vi "ReadPoints.vi"(9 "Transform Points In":T2(array[cluster])) -> (1 "Transform Points out":T2(array[cluster]))   [LabVIEW 2017]
uses:
  ReadTextfileColumns.ctl
  AT901 API/Structures/Struct TransformationPoint.ctl
panel:
  in  "Skip Rows":i32
  in  "Abbrechen":bool
  in  "Column 4":T3
  in  "Column 3":T3
  in  "Column 2":T3
  in  "Column1":T3
  out "subarray":string[][](array[string])
  in  "Skip Lines":i32
  in  "stop":bool
  in  "Delimitor Strichpunkt":bool
  in  "Delimitor Leerzeichen":bool
  in  "DelimitorTab":bool
  in  "file path (use dialog)":path=path "C:/Users/Wehner/Desktop/Testfile.txt"
  # "Textfile Laden"
  # "Vorschau:"
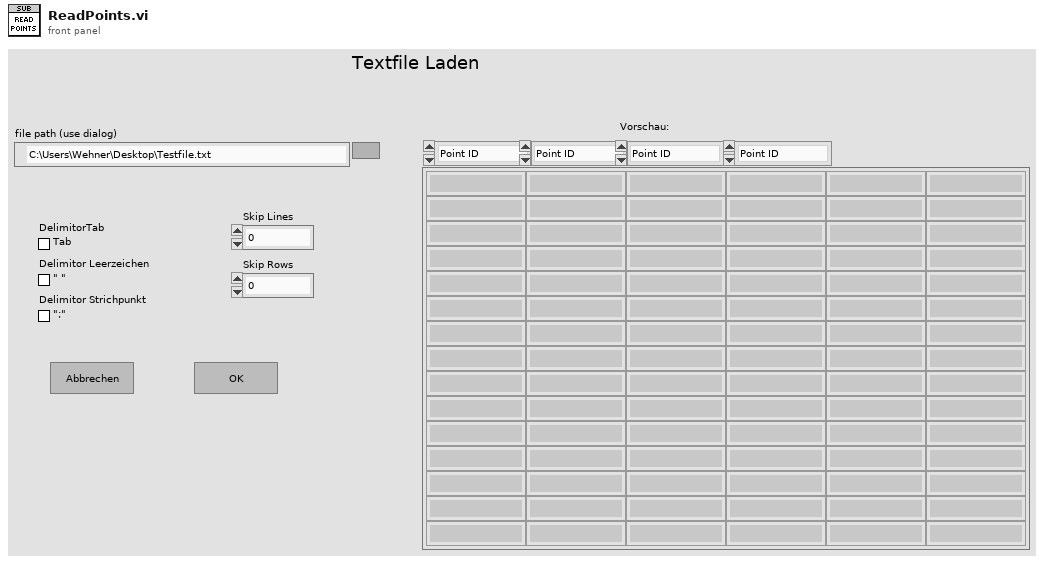
[diagram p1: front panel]
types:
  T1 = typedef "Struct TransformationPoint.ctl" = cluster{"dVal1":dbl, "dVal2":dbl, "dVal3":dbl, "dStd1":dbl, "dStd2":dbl, "dStd3":dbl, "dCovar12":dbl, "dCovar13":dbl, "dCovar23":dbl}
  T2 = cluster{"Punktnummer":string, "Transformation Point":T1}[]
  T3 = typedef "ReadTextfileColumns.ctl" = enum16{"Point ID", "X", "Y", "Z"}
  T4 = cluster{"Punktnummer":string, "Transformation Point":T1}
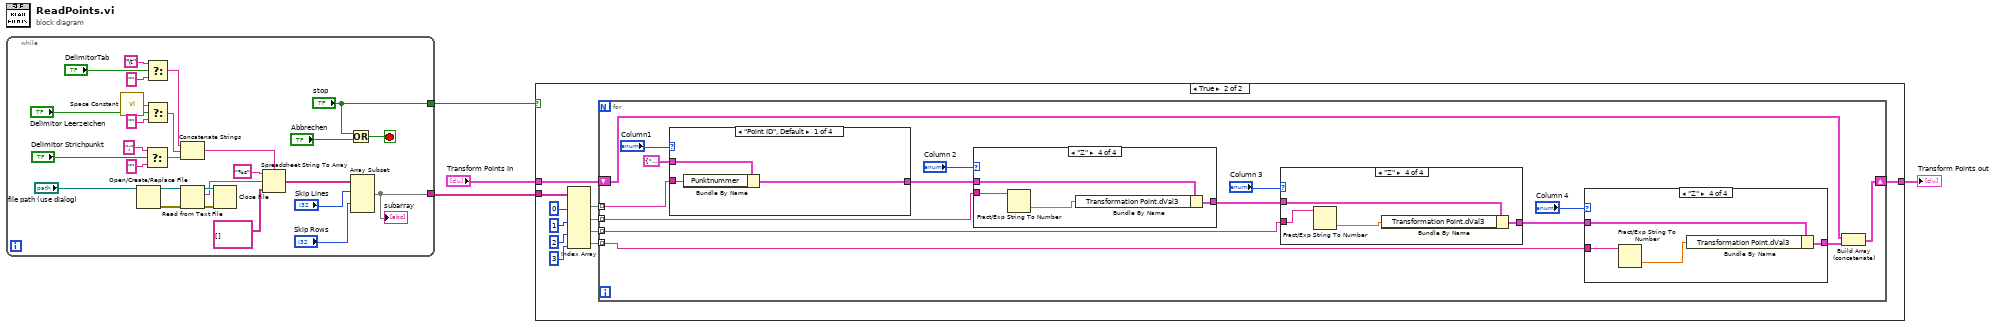
[diagram p0: block diagram]
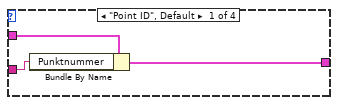
[diagram p3: hidden frame]
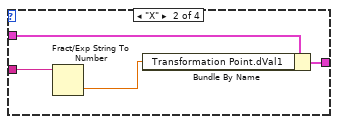
[diagram p4: hidden frame]
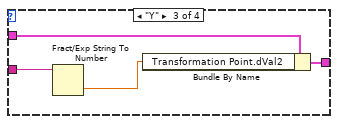
[diagram p5: hidden frame]
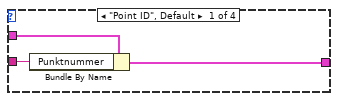
[diagram p6: hidden frame]
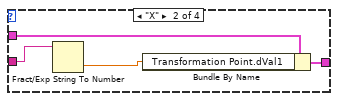
[diagram p7: hidden frame]
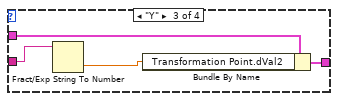
[diagram p8: hidden frame]
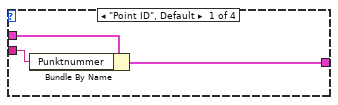
[diagram p9: hidden frame]
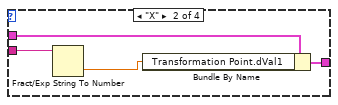
[diagram p10: hidden frame]
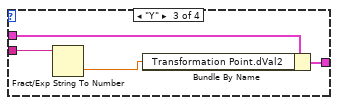
[diagram p11: hidden frame]
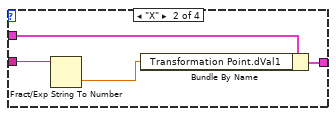
[diagram p12: hidden frame]
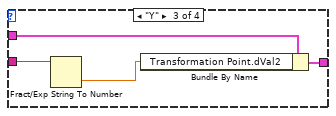
[diagram p13: hidden frame]
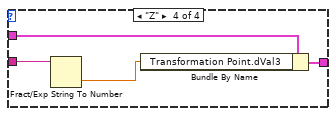
[diagram p14: hidden frame]
diagram:
  n1 = while {
    tunnel: [w15] -> w4
    tunnel: ["stop"] -> w3
    stop <- w13 stop-if-true
    n2 = call <vilib>:"Space Constant.vi"() -> ("String"=w23:string)
    n3 = Open/Create/Replace File(file path (use dialog)="file path (use dialog)") -> (refnum out=w8:refnum<file>, error out=w7:errorcluster)  [unwired: 5 in, 1 out]
    n4 = Select(t=";", s="Delimitor Strichpunkt", f="") -> (s? t:f=w20:string)
    n5 = Select(t="\t", s="DelimitorTab", f="") -> (s? t:f=w18:string)
    n6 = Select(t=w23, s="Delimitor Leerzeichen", f="") -> (s? t:f=w19:string)
    n7 = Concatenate Strings(w18, w19, w20) -> (w27:string)
    n8 = Read from Text File(file (use dialog)=w8, error in=w7) -> (refnum out=w9:refnum<file>, text=w6:string, error out=w10:errorcluster)  [unwired: 2 in, 1 out]
    n9 = Close File(refnum=w9, error in=w10) -> ()  [unwired: 2 out]
    n10 = Spreadsheet String To Array(delimiter (Tab)=w27, format string="%s", spreadsheet string=w6, array type (2D Dbl)=string[][] []) -> (array=w16:string[][])
    n11 = Or(x="stop", y="Abbrechen") -> (x .or. y?=w13:bool)
    n12 = Array Subset(array=w16, index (row)="Skip Lines", index (col)="Skip Rows") -> (w15:string[][])  [unwired: 2 in]
    "subarray" <- w15
  }
  n13 = case shown="True" w3 {
    tunnel: w4 -> [_ w44]
    tunnel: [w33 w34] -> w2
    tunnel: "Transform Points In" -> [w33 w35]
    frame False {
    }
    frame True {
      n14 = Index Array(array=w44, index (col) #1=0 ("disabled index (col)"), index (col) #2=1 ("index (col)"), index (col) #3=2 ("index (col)"), index (col) #4=3 ("index (col)")) -> (element #1=w43:string[], element #2=w38:string[], element #3=w37:string[], element #4=w36:string[])  [unwired: 4 in]
      n15 = for {
        tunnel: w43 -> [w58] mode=indexing
        tunnel: w38 -> [w55] mode=indexing
        tunnel: w37 -> [w52] mode=indexing
        tunnel: w36 -> [w49] mode=indexing
        shift-right: [w45] -> w34
        shift-left: w35 -> [w47]
        n16 = case shown="\"Point ID\", Default" "Column1" {
          tunnel: w58 -> [w107 w111 w112 w116]
          tunnel: [w105 w109 w113 w118] -> w56
          tunnel: T4 {"Punktnummer"="", "Transformation Point"={"dVal1"=0.0, "dVal2"=0.0, "dVal3"=0.0, "dStd1"=0.0, "dStd2"=0.0, "dStd3"=0.0, "dCovar12"=0.0, "dCovar13"=0.0, "dCovar23"=0.0}} ("Actual Point") -> [w106 w108 w114 w117]
          frame "Point ID", Default {
            n17 = Bundle By Name(cluster=w106, "Punktnummer"=w107) -> (w105:T4)
          }
          frame "X" {
            n18 = Fract/Exp String To Number(string=w111) -> (number=w110:dbl)  [unwired: 3 in, 1 out]
            n19 = Bundle By Name(cluster=w108, "Transformation Point.dVal1"=w110) -> (w109:T4)
          }
          frame "Y" {
            n20 = Fract/Exp String To Number(string=w112) -> (number=w115:dbl)  [unwired: 3 in, 1 out]
            n21 = Bundle By Name(cluster=w114, "Transformation Point.dVal2"=w115) -> (w113:T4)
          }
          frame "Z" {
            n22 = Fract/Exp String To Number(string=w116) -> (number=w119:dbl)  [unwired: 3 in, 1 out]
            n23 = Bundle By Name(cluster=w117, "Transformation Point.dVal3"=w119) -> (w118:T4)
          }
        }
        n24 = case shown="\"Z\"" "Column 2" {
          tunnel: [w91 w95 w98 w103] -> w51
          tunnel: w56 -> [w92 w94 w99 w102]
          tunnel: w55 -> [w90 w93 w97 w101]
          frame "Point ID", Default {
            n25 = Bundle By Name(cluster=w92, "Punktnummer"=w90) -> (w91:T4)
          }
          frame "X" {
            n26 = Fract/Exp String To Number(string=w93) -> (number=w96:dbl)  [unwired: 3 in, 1 out]
            n27 = Bundle By Name(cluster=w94, "Transformation Point.dVal1"=w96) -> (w95:T4)
          }
          frame "Y" {
            n28 = Fract/Exp String To Number(string=w97) -> (number=w100:dbl)  [unwired: 3 in, 1 out]
            n29 = Bundle By Name(cluster=w99, "Transformation Point.dVal2"=w100) -> (w98:T4)
          }
          frame "Z" {
            n30 = Fract/Exp String To Number(string=w101) -> (number=w104:dbl)  [unwired: 3 in, 1 out]
            n31 = Bundle By Name(cluster=w102, "Transformation Point.dVal3"=w104) -> (w103:T4)
          }
        }
        n32 = case shown="\"Z\"" "Column 3" {
          tunnel: [w76 w80 w83 w88] -> w50
          tunnel: w51 -> [w77 w79 w84 w87]
          tunnel: w52 -> [w75 w78 w82 w86]
          frame "Point ID", Default {
            n33 = Bundle By Name(cluster=w77, "Punktnummer"=w75) -> (w76:T4)
          }
          frame "X" {
            n34 = Fract/Exp String To Number(string=w78) -> (number=w81:dbl)  [unwired: 3 in, 1 out]
            n35 = Bundle By Name(cluster=w79, "Transformation Point.dVal1"=w81) -> (w80:T4)
          }
          frame "Y" {
            n36 = Fract/Exp String To Number(string=w82) -> (number=w85:dbl)  [unwired: 3 in, 1 out]
            n37 = Bundle By Name(cluster=w84, "Transformation Point.dVal2"=w85) -> (w83:T4)
          }
          frame "Z" {
            n38 = Fract/Exp String To Number(string=w86) -> (number=w89:dbl)  [unwired: 3 in, 1 out]
            n39 = Bundle By Name(cluster=w87, "Transformation Point.dVal3"=w89) -> (w88:T4)
          }
        }
        n40 = case shown="\"Z\"" "Column 4" {
          tunnel: [w61 w65 w68 w73] -> w46
          tunnel: w50 -> [w62 w64 w69 w72]
          tunnel: w49 -> [w60 w63 w67 w71]
          frame "Point ID", Default {
            n41 = Bundle By Name(cluster=w62, "Punktnummer"=w60) -> (w61:T4)
          }
          frame "X" {
            n42 = Fract/Exp String To Number(string=w63) -> (number=w66:dbl)  [unwired: 3 in, 1 out]
            n43 = Bundle By Name(cluster=w64, "Transformation Point.dVal1"=w66) -> (w65:T4)
          }
          frame "Y" {
            n44 = Fract/Exp String To Number(string=w67) -> (number=w70:dbl)  [unwired: 3 in, 1 out]
            n45 = Bundle By Name(cluster=w69, "Transformation Point.dVal2"=w70) -> (w68:T4)
          }
          frame "Z" {
            n46 = Fract/Exp String To Number(string=w71) -> (number=w74:dbl)  [unwired: 3 in, 1 out]
            n47 = Bundle By Name(cluster=w72, "Transformation Point.dVal3"=w74) -> (w73:T4)
          }
        }
        n48 = Build Array (concatenate)(w47, w46) -> (w45:T2)
      }
    }
  }
  "Transform Points out" <- w2
